vi "Create Boundary or Navigation Path.vi"   [LabVIEW 2011]
uses:
  _GlobalVariables&Libraries/ATV Program Global Variables.vi
types:
  T1 = cluster{"End ATV Program":bool, "E-Stop":bool, "Save Logfile":bool, "Logfile Iteration Delay (ms)":u32, "Loop iteration time (ms)":u32, "Logfile Location":path, "Default GPS Navigation Path":path, "Computer":string, "Default GPS Boundary Path":path}
  T2 = cluster{"X":dbl, "Y":dbl, "Zoom":sgl, "Map Type":string, "Google Maps API Key":string, "Map Refresh Rate (ms)":u32, "Navigation Path Color":u32, "Navigation Path Weight":i32, "URL":string, "Boundary Coordinates":cluster{"Latitude":dbl, "Longitude":dbl}[], "GPS Balloon Character":string, "Boundary Path Color":u32, "Boundary Path Weight":i32, "GPS Balloon Size":string, "GPS Balloon Color":string, "GPS Path Color":u32, "GPS Path Weight":i32, "Disable Google Maps":bool}
  T3 = cluster{"Navigation Coordinates":cluster{"Latitude":dbl, "Longitude":dbl}[], "Coordinate Count":u32, "Drive Speed":string, "Steer Angle":dbl, "Steering":dbl, "Direction to next Coordinate":dbl, "Drive":dbl, "Navigation Path":string}
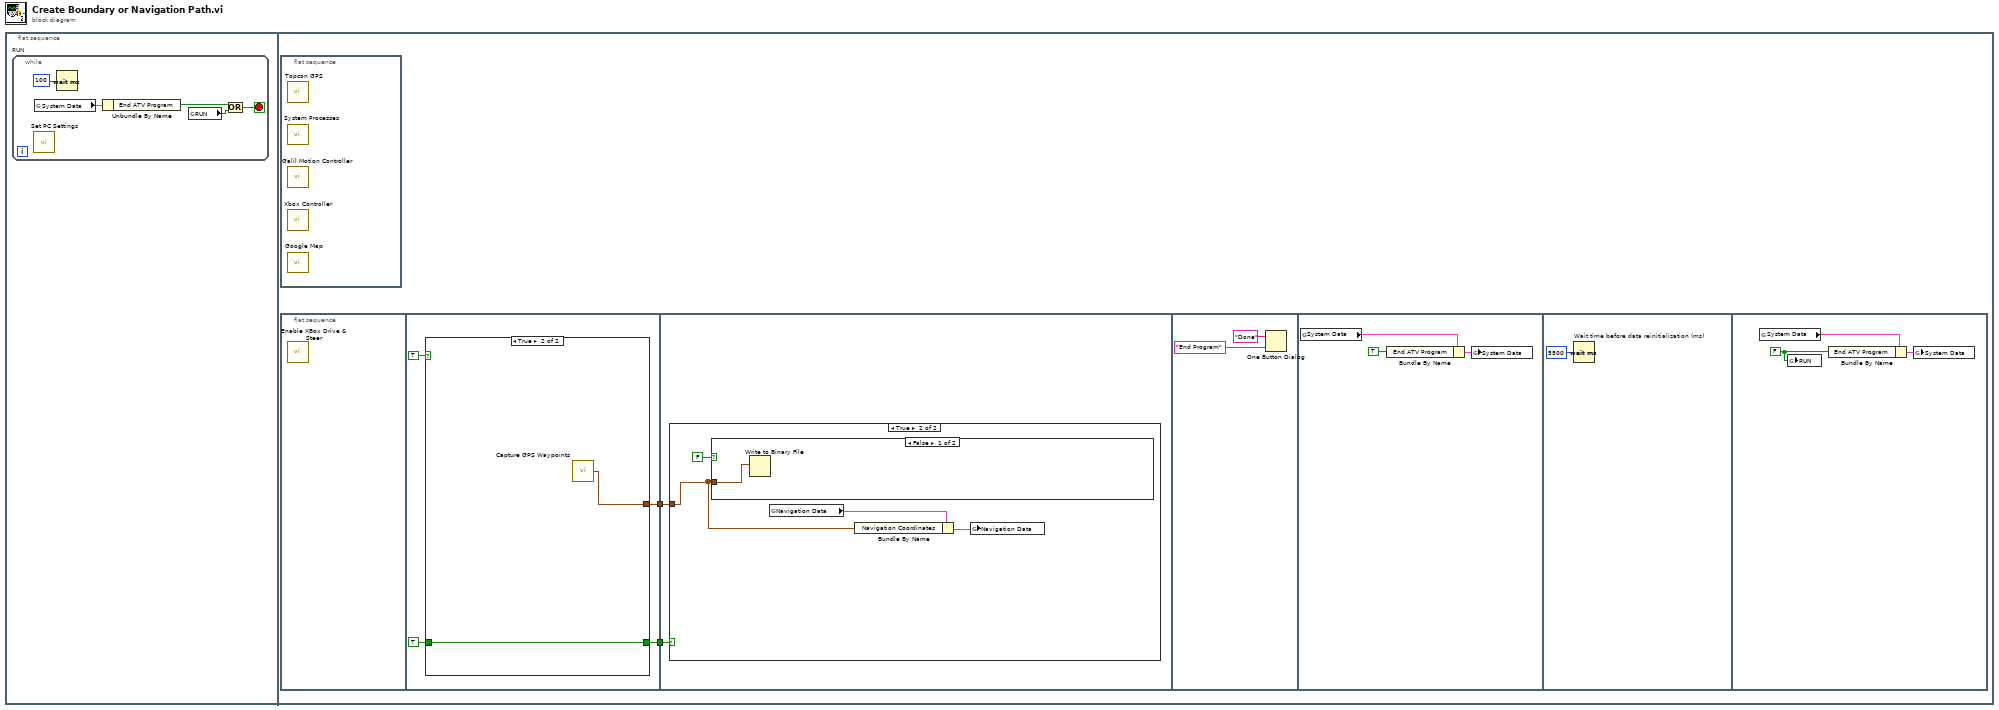
[diagram p0: block diagram]
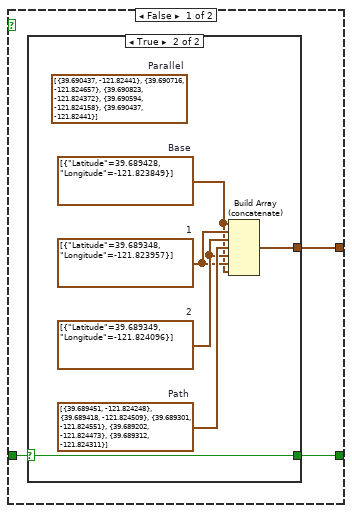
[diagram p2: hidden frame]
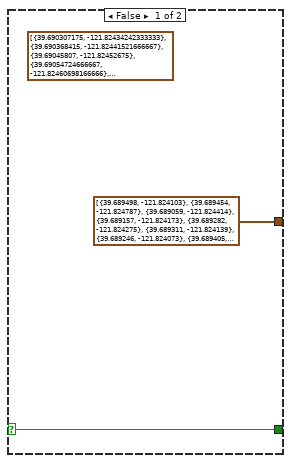
[diagram p3: hidden frame]
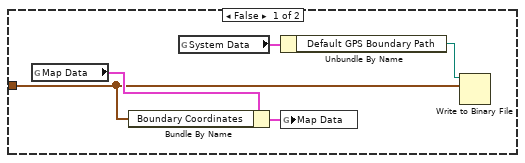
[diagram p4: hidden frame]
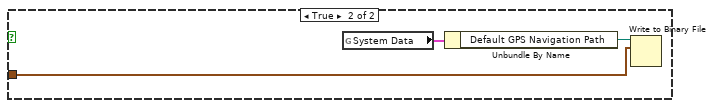
[diagram p5: hidden frame]
diagram:
  n1 = flat-sequence {
    frame #0 {
      n2 = while "RUN" {
        stop <- w1 stop-if-true
        n3 = call "Set PC Settings.vi"() -> ()  [unwired: 12 in]
        n4 = global read "ATV Program Global Variables.vi" "System Data"() -> (w4:T1)
        n5 = Wait (ms)(milliseconds to wait=u32 100) -> ()  [unwired: 1 out]
        n6 = Unbundle By Name(w4) -> ("End ATV Program"=w2:bool)
        n7 = global read "ATV Program Global Variables.vi" "RUN"() -> (w3:bool)
        n8 = Or(x=w2, y=w3) -> (x .or. y?=w1:bool)
      }
    }
    frame #1 {
      n9 = flat-sequence {
        frame #0 {
          n10 = call "Topcon GPS.vi"() -> ()  [unwired: 12 in]
          n11 = call "System Processes.vi"() -> ()  [unwired: 12 in]
          n12 = call "Galil Motion Controller.vi"() -> ()  [unwired: 1 in]
          n13 = call "Xbox Controller.vi"() -> ()  [unwired: 1 in]
          n14 = call "Google Map.vi"() -> ()  [unwired: 1 in]
        }
      }
      n15 = flat-sequence {
        tunnel: [w11] -> w7
        tunnel: [w9] -> w6
        tunnel: w7 -> [w26]
        tunnel: w6 -> [w25]
        frame #0 {
          n16 = call "Enable XBox Drive & Steer.vi"() -> ()  [unwired: 12 in]
        }
        frame #1 {
          n17 = case shown="True" TRUE {
            tunnel: [w14 w23] -> w11
            tunnel: [w13 w24] -> w9
            tunnel: TRUE ("Boolean") -> [w12 w24]
            frame False {
              n18 = case shown="True" w12 {
                selector: w12 -> [w16 w22]
                tunnel: [cluster{"Latitude":dbl, "Longitude":dbl}[] [{"Latitude"=39.689498, "Longitude"=-121.824103}, {"Latitude"=39.689454, "Longitude"=-121.824787}, {"Latitude"=39.689059, "Longitude"=-121.824414}, {"Latitude"=39.689157, "Longitude"=-121.824173}, {"Latitude"=39.689282, "Longitude"=-121.824275}, {"Latitude"=39.689311, "Longitude"=-121.824139}, {"Latitude"=39.689246, "Longitude"=-121.824073}, {"Latitude"=39.689405, "Longitude"=-121.82376}, {"Latitude"=39.689469, "Longitude"=-121.823831}, {"Latitude"=39.68938, "Longitude"=-121.823981}] ("Navigation Coordinates") w17] -> w14
                tunnel: [w16 w22] -> w13
                frame False {
                  (unwired) cluster{"Latitude":dbl, "Longitude":dbl}[] [{"Latitude"=39.690307175, "Longitude"=-121.82434242333333}, {"Latitude"=39.690368415, "Longitude"=-121.82441521666667}, {"Latitude"=39.69045807, "Longitude"=-121.82452675}, {"Latitude"=39.69054724666667, "Longitude"=-121.82460698166666}, {"Latitude"=39.69054724666667, "Longitude"=-121.82460698166666}, {"Latitude"=39.69066610833333, "Longitude"=-121.82466573666666}, {"Latitude"=39.69075449333333, "Longitude"=-121.82466967166667}, {"Latitude"=39.690855383333336, "Longitude"=-121.82454980833333}, {"Latitude"=39.69091665166667, "Longitude"=-121.82438014833333}, {"Latitude"=39.690999696666665, "Longitude"=-121.82420006666666}, {"Latitude"=39.691041096666666, "Longitude"=-121.82408576833333}, {"Latitude"=39.690981783333335, "Longitude"=-121.82387681}, {"Latitude"=39.690966295, "Longitude"=-121.823736075}, {"Latitude"=39.69086914166667, "Longitude"=-121.823745275}, {"Latitude"=39.69076178833333, "Longitude"=-121.82392718166666}, {"Latitude"=39.69065429333333, "Longitude"=-121.82408263333333}, {"Latitude"=39.69049326333333, "Longitude"=-121.82406832666666}, {"Latitude"=39.690326703333334, "Longitude"=-121.824279895}] ("Navigation Coordinates")
                }
                frame True {
                  w21 = cluster{"Latitude":dbl, "Longitude":dbl}[] [{"Latitude"=39.689451, "Longitude"=-121.824248}, {"Latitude"=39.689418, "Longitude"=-121.824509}, {"Latitude"=39.689301, "Longitude"=-121.824551}, {"Latitude"=39.689202, "Longitude"=-121.824473}, {"Latitude"=39.689312, "Longitude"=-121.824311}]  # Path
                  w20 = cluster{"Latitude":dbl, "Longitude":dbl}[] [{"Latitude"=39.689349, "Longitude"=-121.824096}]  # 2
                  w19 = cluster{"Latitude":dbl, "Longitude":dbl}[] [{"Latitude"=39.689348, "Longitude"=-121.823957}]  # 1
                  w18 = cluster{"Latitude":dbl, "Longitude":dbl}[] [{"Latitude"=39.689428, "Longitude"=-121.823849}]  # Base
                  (unwired) cluster{"Latitude":dbl, "Longitude":dbl}[] [{"Latitude"=39.690437, "Longitude"=-121.82441}, {"Latitude"=39.690716, "Longitude"=-121.824657}, {"Latitude"=39.690823, "Longitude"=-121.824372}, {"Latitude"=39.690594, "Longitude"=-121.824158}, {"Latitude"=39.690437, "Longitude"=-121.82441}]  # Parallel
                  n19 = Build Array (concatenate)(w18, w19, w20, w21, w20, w19, w18) -> (w17:cluster{"Latitude":dbl, "Longitude":dbl}[])
                }
              }
            }
            frame True {
              n20 = call "Capture GPS Waypoints.vi"() -> ("GPS Coordinates"=w23:cluster{"Latitude":dbl, "Longitude":dbl}[])
            }
          }
        }
        frame #2 {
          n21 = case shown="True" w25 {
            tunnel: w26 -> [w28 w33]
            frame False {
              n22 = global read "ATV Program Global Variables.vi" "Map Data"() -> (w29:T2)
              n23 = Bundle By Name(cluster=w29, "Boundary Coordinates"=w28) -> (w30:T2)
              n24 = global read "ATV Program Global Variables.vi" "System Data"() -> (w27:T1)
              n25 = Unbundle By Name(w27) -> ("Default GPS Boundary Path"=w31:path)
              n26 = global write "ATV Program Global Variables.vi" "Map Data"(w30) -> ()
              n27 = Write to Binary File(file (use dialog)=w31, data=w28) -> ()  [unwired: 4 in, 3 out]
            }
            frame True {
              n28 = case shown="False" FALSE {
                tunnel: w33 -> [w36 w37]
                frame False {
                  n29 = Write to Binary File(data=w36) -> ()  [unwired: 5 in, 3 out]
                }
                frame True {
                  n30 = global read "ATV Program Global Variables.vi" "System Data"() -> (w38:T1)
                  n31 = Unbundle By Name(w38) -> ("Default GPS Navigation Path"=w39:path)
                  n32 = Write to Binary File(file (use dialog)=w39, data=w37) -> ()  [unwired: 4 in, 3 out]
                }
              }
              n33 = global read "ATV Program Global Variables.vi" "Navigation Data"() -> (w34:T3)
              n34 = Bundle By Name(cluster=w34, "Navigation Coordinates"=w33) -> (w35:T3)
              n35 = global write "ATV Program Global Variables.vi" "Navigation Data"(w35) -> ()
            }
          }
        }
        frame #3 {
          n36 = One Button Dialog(message="Done", button name ("OK")="End Program") -> ()  [unwired: 1 out]
        }
        frame #4 {
          n37 = global read "ATV Program Global Variables.vi" "System Data"() -> (w44:T1)
          n38 = Bundle By Name(cluster=w44, "End ATV Program"=TRUE ("End Program")) -> (w43:T1)
          n39 = global write "ATV Program Global Variables.vi" "System Data"(w43) -> ()
        }
        frame #5 {
          n40 = Wait (ms) "Wait time before data reinitialization (ms)"(milliseconds to wait=u32 5500) -> ()  [unwired: 1 out]
        }
        frame #6 {
          w46 = FALSE ("End Program")
          n41 = global read "ATV Program Global Variables.vi" "System Data"() -> (w48:T1)
          n42 = global write "ATV Program Global Variables.vi" "RUN"(w46) -> ()
          n43 = Bundle By Name(cluster=w48, "End ATV Program"=w46) -> (w47:T1)
          n44 = global write "ATV Program Global Variables.vi" "System Data"(w47) -> ()
        }
      }
    }
  }
